vi "April Tag Compute Offset Angle.vi"(9 "Internal Parameters":T1, 11 "Tag Center":cluster{"X (cu)":dbl, "Y":dbl}) -> (3 "Bearing":dbl=569.258018632146)   [LabVIEW 2025]
uses:
  <vilib>/vision/Calibration.llb/Internal Parameters.ctl
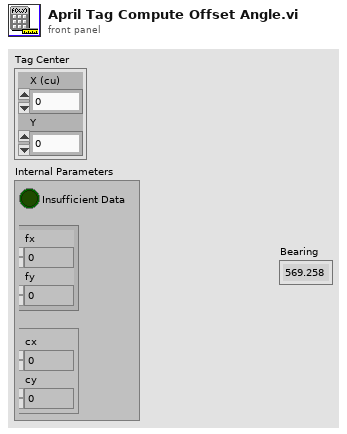
[diagram p1: front panel]
types:
  T1 = typedef "Internal Parameters.ctl" = cluster{"Insufficient Data":bool, "Focal Length (pixel)":cluster{"fx":sgl, "fy":sgl}, "Optical Center (pixel)":cluster{"cx":sgl, "cy":sgl}}
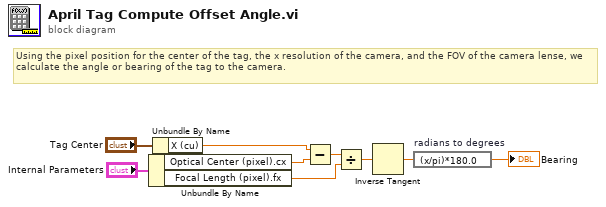
[diagram p0: block diagram]
diagram:
  # "Using the pixel position for the center of the tag, the x resolution of the camera, and the FOV of the camera lense, we calculate the angle or bearing of the tag to the camera."
  n1 = Unbundle By Name("Internal Parameters") -> ("Optical Center (pixel).cx"=w6:sgl, "Focal Length (pixel).fx"=w4:sgl)
  n2 = Unbundle By Name("Tag Center") -> ("X (cu)"=w1:dbl)
  n3 = Subtract(x=w1, y=w6) -> (x-y=w5:dbl)
  n4 = Divide(x=w5, y=w4) -> (x/y=w3:dbl)
  n5 = Inverse Tangent(1:w3) -> (0:w7:dbl)
  n6 = expression code="(x/pi)*180.0" "radians to degrees"(w7) -> (→"Bearing":dbl)
